vi "insertStack.vi"(7 "error in (no error)":errorcluster, 8 "novo elemento":T1={"up"=2.0, "down"=1.0}, 9 "pilha input":T1[](array[typedef]), 10 "Utilities in":refnum<class "Utilities.lvclass">) -> (0 "error out":errorcluster, 2 "pilha output":T1[](array[typedef]), 3 "Utilities out":refnum<class "Utilities.lvclass">)   [LabVIEW 2023, in "Utilities.lvclass"]
uses:
  Utilities.lvclass
  segment.ctl
  Utilities.lvclass/Utilities.ctl
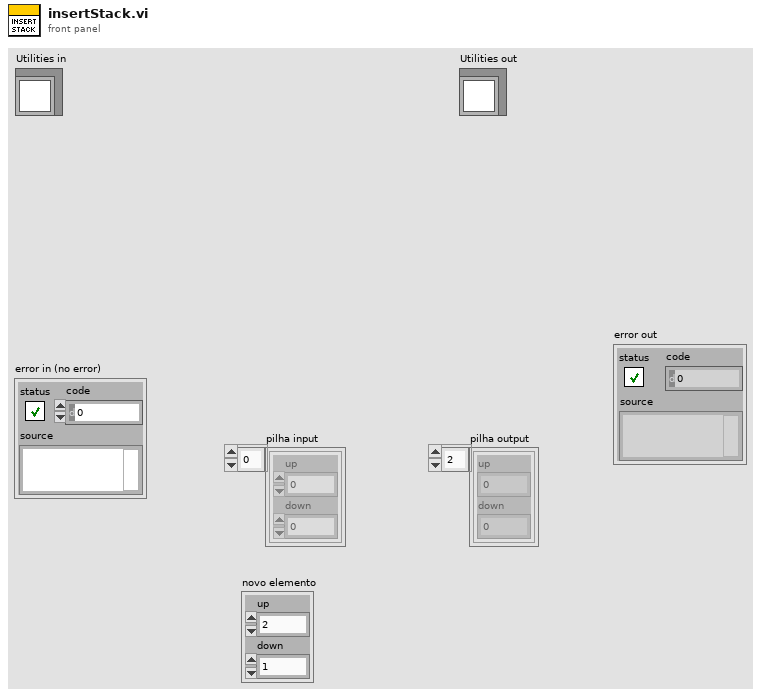
[diagram p1: front panel]
types:
  T1 = typedef "Utilities.lvclass/segment.ctl" = cluster{"up":dbl, "down":dbl}
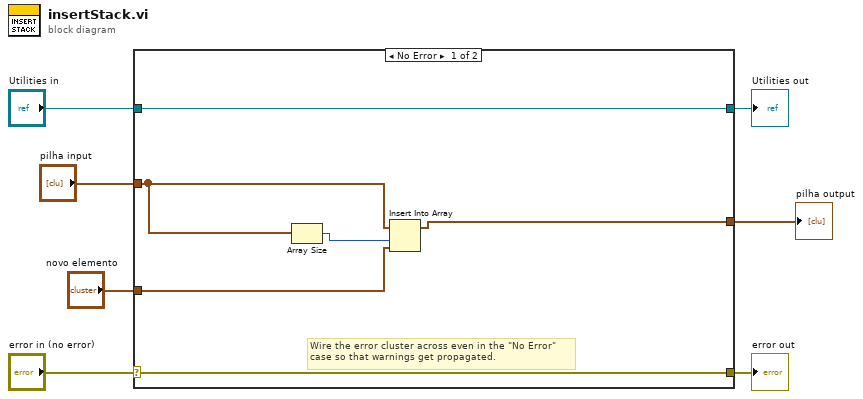
[diagram p0: block diagram]
diagram:
  n1 = case shown="No Error" "error in (no error)" {
    selector: "error in (no error)" -> [w12 w16]
    tunnel: [w12 w16] -> w6
    tunnel: [w13 w15] -> w4
    tunnel: "Utilities in" -> [w13 w15]
    tunnel: "pilha input" -> [w10 w14]
    tunnel: [w9 w14] -> w2
    tunnel: "novo elemento" -> [w8 _]
    frame No Error {
      # "Wire the error cluster across even in the \"No Error\"\ncase so that warnings get propagated."
      n2 = Array Size(array=w10) -> (size(s)=w11:i32)
      n3 = Insert Into Array(array=w10, index=w11, new element=w8) -> (w9:T1[])
    }
    frame Error {
    }
  }
  "error out" <- w6
  "Utilities out" <- w4
  "pilha output" <- w2
